vi "Command Voltages Check.vi"() -> ()   [LabVIEW 2009]
uses:
  lib/Apps/On Off Button.ctl
  lib/Calibration/Command Voltage Check Ramp States.ctl
  Test Utilities/DAQ Read Actions.ctl
  <vilib>/DAQmx/write.llb/DAQmx Write (Analog 1D DBL NChan 1Samp).vi
  Program Files (x86)/National Instruments/LabVIEW 2009/resource/objmgr/daqmx.rc
panel:
  in  "error out":errorcluster
  out "Cmd Volt Chk Ramp States":T1
  in  "Ramping":T2
  in  "Number of\nIntervals":i32
  in  "Half Period (msec)":i32
  in  "Peak Value":dbl
  in  "Offset":dbl
  out "Diffs":dbl[](array[numeric])=[-7.680882880270997, -8.566659800159199, -9.658116593296763, -9.594949810916727, -8.940447035067507, -8.192445315897492] format="%^#_10g"
  out "Write error out":errorcluster
  out "Monitor":dbl[](array[numeric])=[-7.680882880270997, -8.566659800159199, -9.658116593296763, -9.594949810916727, -8.940447035067507, -8.192445315897492] format="%^#_10g"
  out "Command \nVoltage":dbl[](array[numeric])=[-0.0, -0.0, -0.0, -0.0, -0.0, -0.0] format="%^#_10g"
  out "Control Voltage":dbl[](array[numeric])=[-0.0, -0.0, -0.0, -0.0, -0.0, -0.0]
  in  "Quit":bool
  in  "rate":dbl=100.0
  in  "samples per \nchannel":i32=30 caption="samples per channel"
  in  "Command Voltage Task":refnum<k21>="Command Voltage"
  in  "Monitor Task":refnum<k21>="All Readings"
  in  "Actuator":i32(listbox)
  out "Command \nVoltages":T3(graph)={"Average[0]"=-7.17251209904047, "Average[1]"=-8.19396103384171, "Average[2]"=-9.68369051887908, "Average[3]"=-9.45574535938537, "Average[4]"=-9.241187346298316, "Average[5]"=-8.612741694704903, "Average[6]"=0.0, "Average[7]"=0.0, "Average[8]"=0.0}
  out "Monitor":T3(graph)={"Average[0]"=-7.17251209904047, "Average[1]"=-8.19396103384171, "Average[2]"=-9.68369051887908, "Average[3]"=-9.45574535938537, "Average[4]"=-9.241187346298316, "Average[5]"=-8.612741694704903, "Average[6]"=0.0, "Average[7]"=0.0, "Average[8]"=0.0}
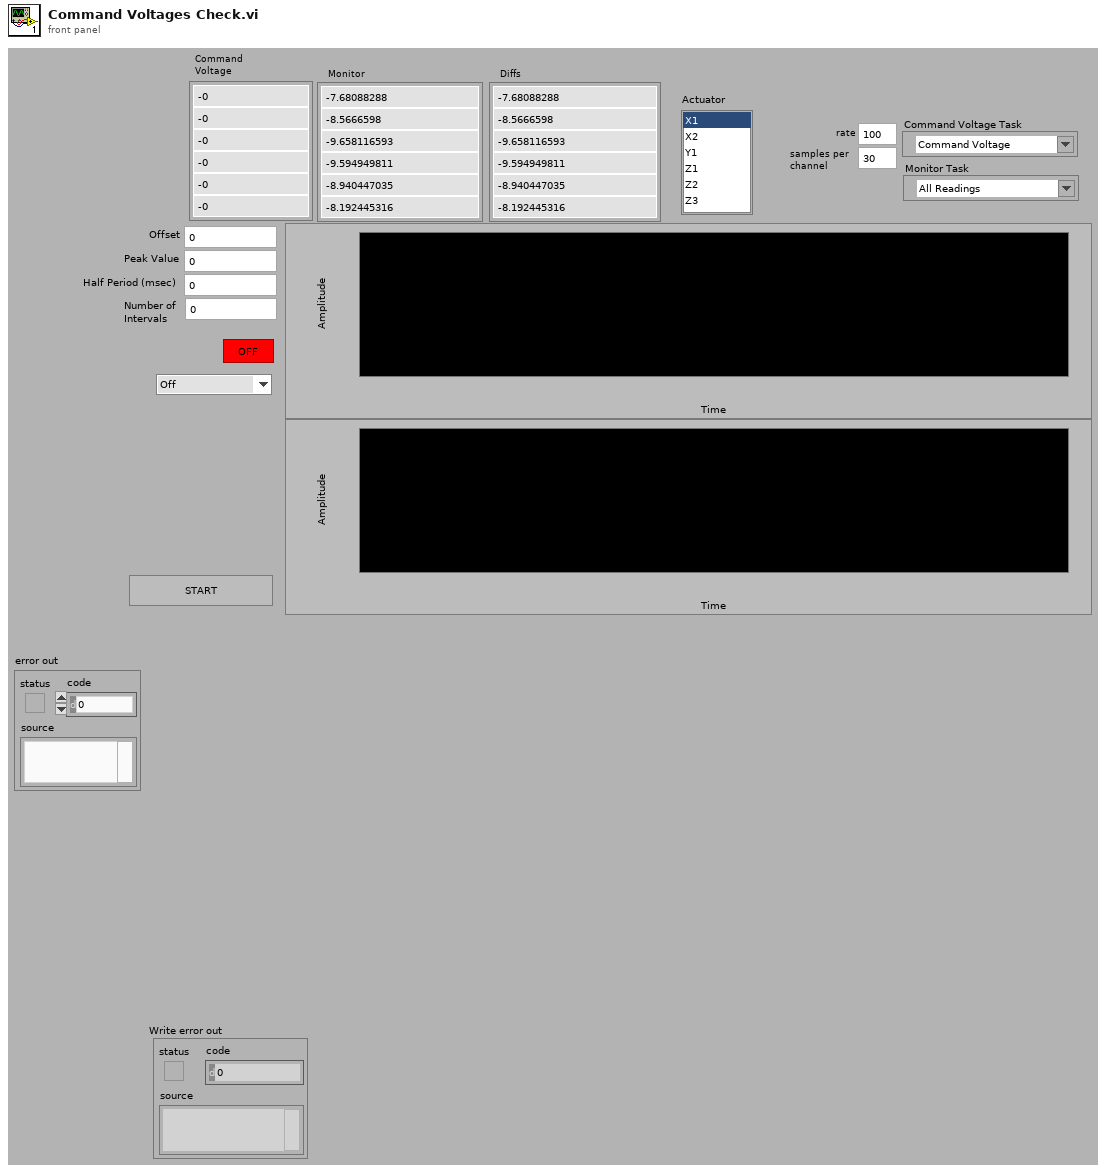
[diagram p1: front panel]
types:
  T1 = typedef "Command Voltage Check Ramp States.ctl" = enum16{"Off", "Start", "Ramp Up", "Ramp Down", "Stop"}
  T2 = typedef "On Off Button.ctl" = bool
  T3 = cluster{"Average[0]":dbl, "Average[1]":dbl, "Average[2]":dbl, "Average[3]":dbl, "Average[4]":dbl, "Average[5]":dbl, "Average[6]":dbl, "Average[7]":dbl, "Average[8]":dbl}
  T4 = typedef "DAQ Read Actions.ctl" = enum16{"Start", "Read", "Stop"}
  T5 = cluster{"Control Voltage[0]":dbl, "Control Voltage[1]":dbl, "Control Voltage[2]":dbl, "Control Voltage[3]":dbl, "Control Voltage[4]":dbl, "Control Voltage[5]":dbl, "Control Voltage[6]":dbl, "Control Voltage[7]":dbl, "Control Voltage[8]":dbl}
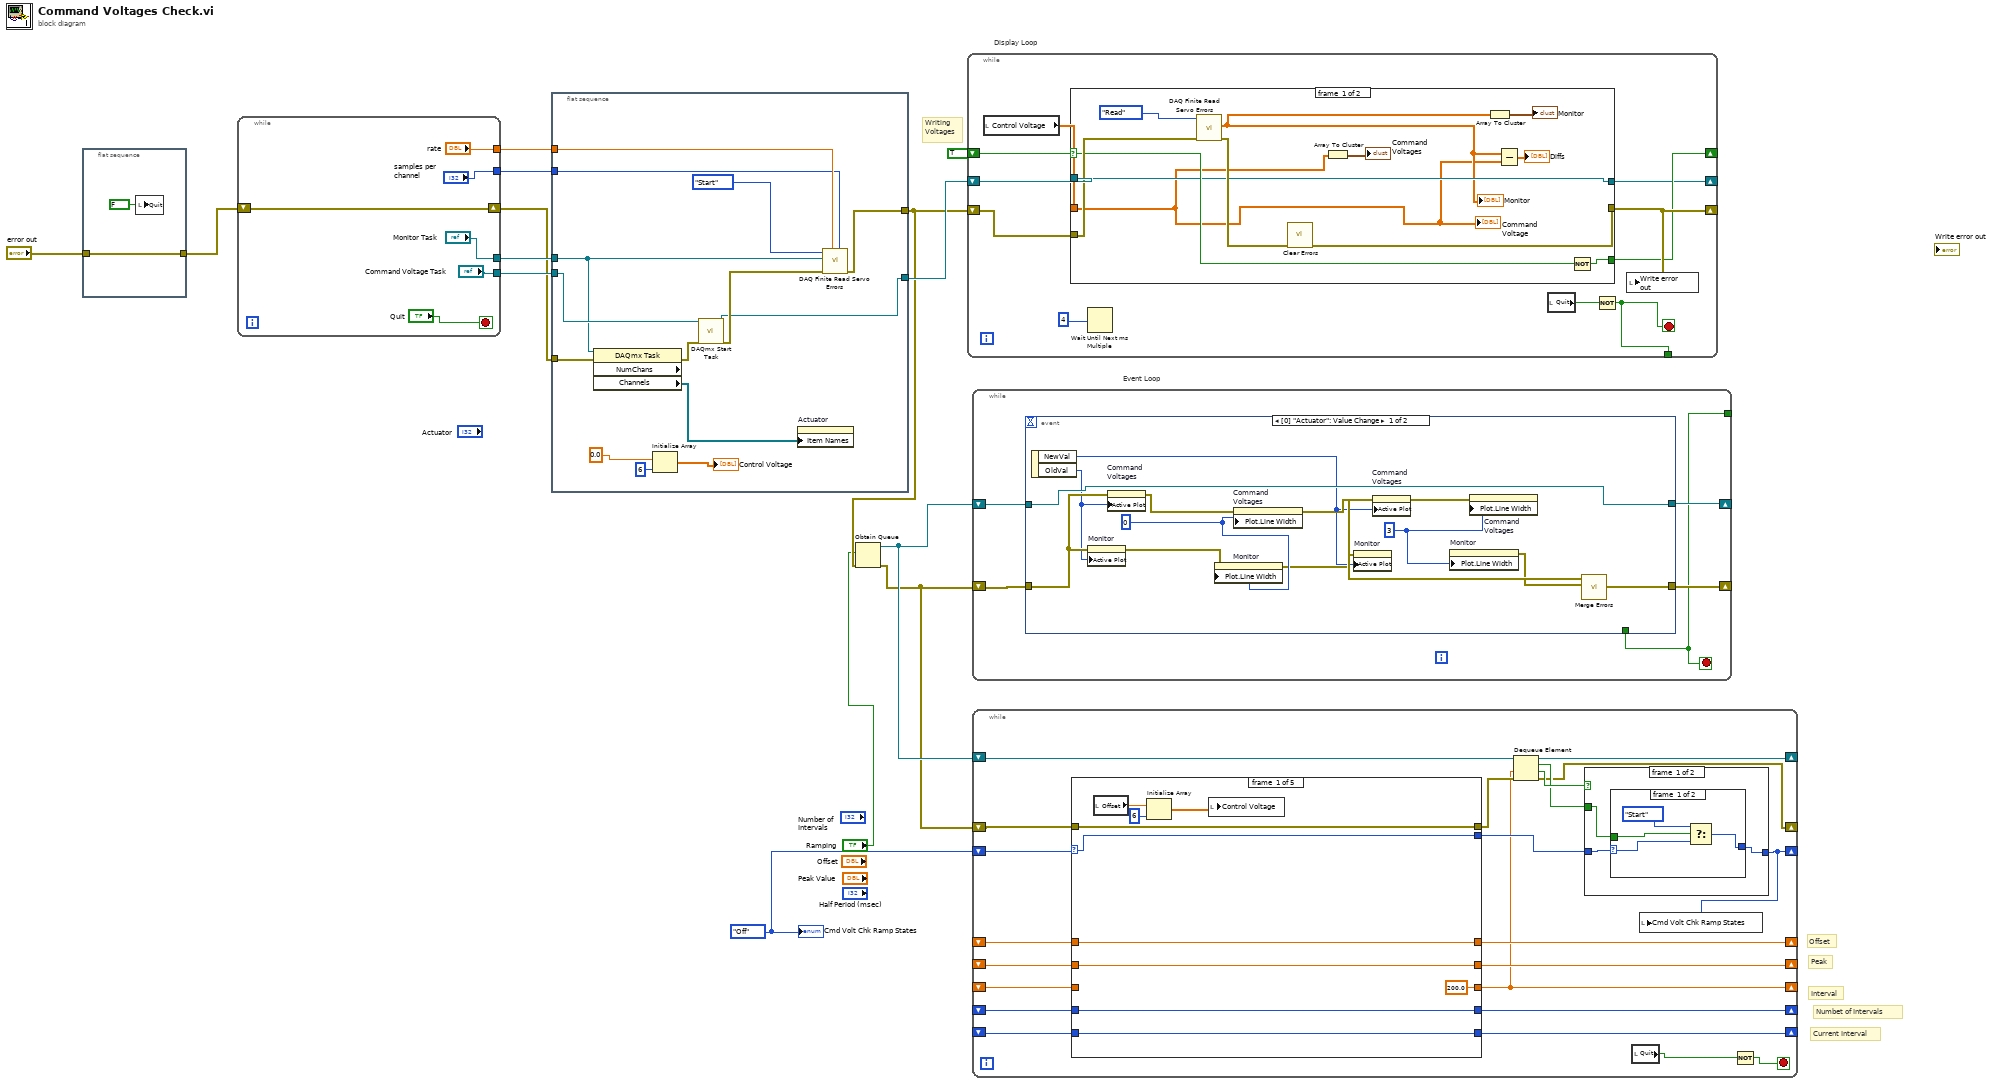
[diagram p0: block diagram]
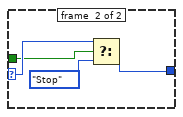
[diagram p2: hidden frame]
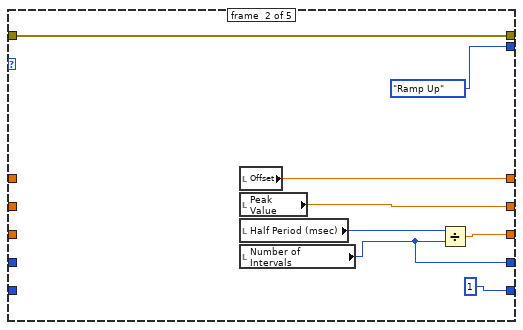
[diagram p4: hidden frame]
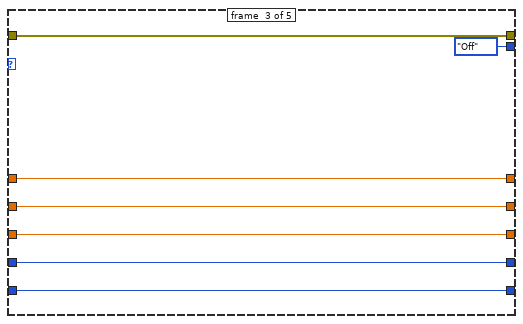
[diagram p5: hidden frame]
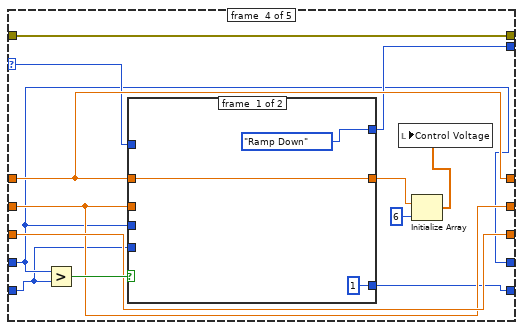
[diagram p6: hidden frame]
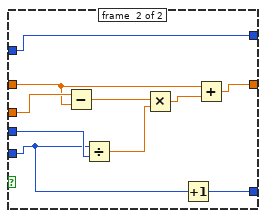
[diagram p7: hidden frame]
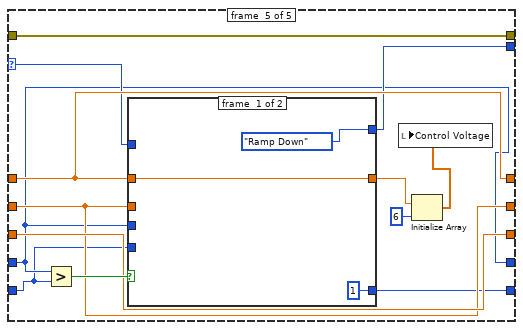
[diagram p8: hidden frame]
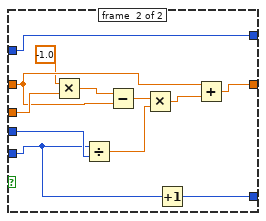
[diagram p9: hidden frame]
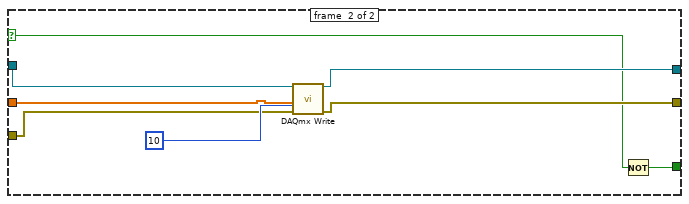
[diagram p10: hidden frame]
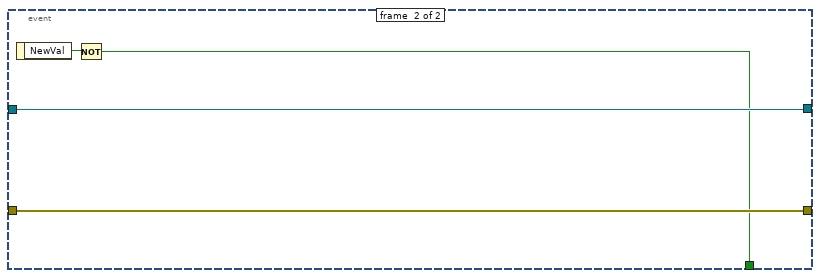
[diagram p11: hidden frame]
diagram:
  w8 = Command_Voltage_Check_Ramp_States."Off" ("Cmd Volt Chk Ramp States")
  # "Current Interval"
  # "Numbet of Intervals"
  # "Interval"
  # "Peak"
  # "Offset"
  # "Writing\nVoltages"
  n1 = flat-sequence {
    tunnel: "error out" -> [w16]
    tunnel: [w16] -> w1
    frame #0 {
      n2 = local write "Quit"(FALSE ("Quit")) -> ()
    }
  }
  n3 = while {
    tunnel: ["Command Voltage Task"] -> w14
    tunnel: ["Monitor Task"] -> w13
    tunnel: ["rate"] -> w12
    tunnel: ["samples per \nchannel"] -> w11
    shift-right: [w17] -> w3
    shift-left: w1 -> [w17]
    stop <- "Quit" stop-if-true
  }
  n4 = flat-sequence {
    tunnel: w14 -> [w35]
    tunnel: w13 -> [w26]
    tunnel: w12 -> [w34]
    tunnel: w11 -> [w33]
    tunnel: [w28] -> w7
    tunnel: [w27] -> w10
    tunnel: w3 -> [w23]
    frame #0 {
      n5 = property class="DAQmx Task" props=["NumChans", "Channels"](reference=w26, error in=w23) -> (error out=w25:errorcluster, "Channels"=w24:refnum<k21>[])  [unwired: 2 out]
      n6 = Initialize Array(0.0, 6 ("dimension size")) -> (→"Control Voltage":dbl[])
      n7 = call <vilib>:"DAQmx Start Task.vi"("task/channels in"=w35, "error in"=w25) -> ("task out"=w27:refnum<k21>, "error out"=w29:errorcluster)  [unwired: 12 out]
      n8 = property on="Actuator" class="LstBox (strict)"("Item Names"=w24) -> ()  [unwired: 2 in, 2 out]
      n9 = call "DAQ Finite Read Servo Errors.vi"("samples per channel"=w33, "rate"=w34, "error in"=w29, "task/channels in"=w26, "Action"=DAQ_Read_Actions."Start") -> ("error out"=w28:errorcluster)  [unwired: 6 out]
    }
  }
  n10 = Obtain Queue(element data type="Ramping", error in (no error)=w7) -> (queue out=w6:refnum<queue>, error out=w4:errorcluster)  [unwired: 3 in, 1 out]
  n11 = while "Display Loop" {
    shift-right: [w41] -> _
    shift-left: w7 -> [w42]
    tunnel: [w44] -> _
    shift-right: [w40] -> _
    shift-left: TRUE -> [w39]
    shift-right: [w37] -> _
    shift-left: w10 -> [w38]
    stop <- w44 stop-if-true
    n12 = local read "Control Voltage"() -> (w43:dbl[])
    n13 = case shown="True" w39 {
      selector: w39 -> [w52 w59]
      tunnel: w43 -> [w47 w62]
      tunnel: w42 -> [w55 w64]
      tunnel: [w53 w63] -> w41
      tunnel: [w51 w60] -> w40
      tunnel: w38 -> [w50 w65]
      tunnel: [w50 w61] -> w37
      frame #0 {
        n14 = call "DAQ Finite Read Servo Errors.vi"("error in"=w55, "Action"=DAQ_Read_Actions."Read") -> ("error out"=w54:errorcluster, "Average"=w48:dbl[])  [unwired: 3 in, 5 out]
        "Monitor" <- w48
        n15 = call <vilib>:"Clear Errors.vi"("error in (no error)"=w54) -> ("error out"=w53:errorcluster)  [unwired: 6 out]
        n16 = Array To Cluster(array=w47) -> (cluster=→"Command \nVoltages":T5)
        n17 = Array To Cluster(array=w48) -> (cluster=→"Monitor":T3)
        n18 = Subtract(x=w48, y=w47) -> (x-y=→"Diffs":dbl[])
        n19 = Not(x=w52) -> (.not. x?=w51:bool)
        "Command \nVoltage" <- w47
      }
      frame #1 {
        n20 = call-poly <vilib>:"DAQmx Write.vi"("task/channels in"=w65, "data"=w62, "timeout"=10, "error in"=w64) -> ("task out"=w61:refnum<k21>, "error out"=w63:errorcluster)  [unwired: 1 in, 9 out]
        n21 = Not(x=w59) -> (.not. x?=w60:bool)
      }
    }
    n22 = Wait Until Next ms Multiple(millisecond multiple=4) -> ()  [unwired: 1 out]
    n23 = local read "Quit"() -> (w45:bool)
    n24 = Not(x=w45) -> (.not. x?=w44:bool)
    n25 = local write "Write error out"(w41) -> ()
  }
  n26 = while "Event Loop" {
    tunnel: [w67] -> _
    shift-right: [w68] -> _
    shift-left: w4 -> [w70]
    shift-right: [w69] -> _
    shift-left: w6 -> [w71]
    stop <- w67 stop-if-true
    n27 = event shown="[0] \"Actuator\": Value Change" {
      selector: _ -> [_ _]
      dyn-events: _ -> [_ _]
      timeout: _ -> [_ _]
      tunnel: w71 -> [w81 w88]
      tunnel: w70 -> [w80 w89]
      tunnel: [w81 w88] -> w69
      tunnel: [w73 w89] -> w68
      tunnel: [_ w86] -> w67
      event #0 {
        w74 = u8 3 ("Plot.Line Width")
        w78 = u8 0 ("Plot.Line Width")
        n28 = event-data() -> ("NewVal"=w75:i32, "OldVal"=w79:i32)  [unwired: 1 out]
        n29 = property on="Monitor" class="WFChart (strict)"(error in=w80, "Active Plot"=w79) -> (error out=w77:errorcluster)  [unwired: 1 in, 1 out]
        n30 = property on="Command \nVoltages" class="WFChart (strict)"(error in=w80, "Active Plot"=w79) -> (error out=w85:errorcluster)  [unwired: 1 in, 1 out]
        n31 = property on="Monitor" class="WFChart (strict)"(error in=w77, "Plot.Line Width"=w78) -> (error out=w76:errorcluster)  [unwired: 1 in, 1 out]
        n32 = property on="Command \nVoltages" class="WFChart (strict)"(error in=w85, "Plot.Line Width"=w78) -> (error out=w84:errorcluster)  [unwired: 1 in, 1 out]
        n33 = property on="Monitor" class="WFChart (strict)"(error in=w76, "Active Plot"=w75) -> ()  [unwired: 1 in, 2 out]
        n34 = property on="Command \nVoltages" class="WFChart (strict)"(error in=w84, "Active Plot"=w75) -> (error out=w83:errorcluster)  [unwired: 1 in, 1 out]
        n35 = property on="Monitor" class="WFChart (strict)"("Plot.Line Width"=w74) -> (error out=w72:errorcluster)  [unwired: 2 in, 1 out]
        n36 = property on="Command \nVoltages" class="WFChart (strict)"(error in=w83, "Plot.Line Width"=w74) -> (error out=w82:errorcluster)  [unwired: 1 in, 1 out]
        n37 = call <vilib>:"Merge Errors.vi"("error in 2 (no error)"=w72, "error in 1 (no error)"=w82) -> ("error out"=w73:errorcluster)  [unwired: 5 in]
      }
      event #1 {
        n38 = event-data() -> ("NewVal"=w87:bool)  [unwired: 1 out]
        n39 = Not(x=w87) -> (.not. x?=w86:bool)
      }
    }
  }
  n40 = while {
    shift-right: [w93] -> _
    shift-left: w8 -> [w111]
    shift-right: [w104] -> _
    shift-left: w4 -> [w110]
    shift-right: [w103] -> _
    shift-left: w6 -> [w109]
    shift-right: [w92] -> _
    shift-left: _ -> [w96]
    shift-right: [w101] -> _
    shift-left: _ -> [w97]
    shift-right: [w102] -> _
    shift-left: _ -> [w98]
    shift-right: [w100] -> _
    shift-left: _ -> [w95]
    shift-right: [w99] -> _
    shift-left: _ -> [w94]
    stop <- w91 stop-if-true
    n41 = case shown="\"Off\"" w111 {
      selector: w111 -> [w129 _ _ w153 w179]
      tunnel: w110 -> [w130 w134 w143 w161 w187]
      tunnel: [w130 w134 w143 w161 w187] -> w108
      tunnel: [w129 Command_Voltage_Check_Ramp_States."Ramp Up" ("Cmd Volt Chk Ramp States") Command_Voltage_Check_Ramp_States."Off" ("Cmd Volt Chk Ramp States") w152 w178] -> w105
      tunnel: [w128 w141 w148 w155 w181] -> w102
      tunnel: [w127 w140 w147 w154 w180] -> w101
      tunnel: [200.0 w138 w144 w159 w185] -> w92
      tunnel: [w125 w137 w146 w151 w177] -> w100
      tunnel: [w124 1 w145 w149 w175] -> w99
      tunnel: w98 -> [w128 _ w148 w155 w181]
      tunnel: w97 -> [w127 _ w147 w154 w180]
      tunnel: w96 -> [_ _ w144 w159 w185]
      tunnel: w95 -> [w125 _ w146 w151 w177]
      tunnel: w94 -> [w124 _ w145 w150 w176]
      frame #0 {
        n42 = local read "Offset"() -> (w133:dbl)
        n43 = Initialize Array(w133, 6 ("dimension size")) -> (w131:dbl[])
        n44 = local write "Control Voltage"(w131) -> ()
      }
      frame #1 {
        n45 = local read "Offset"() -> (w141:dbl)
        n46 = local read "Peak Value"() -> (w140:dbl)
        n47 = local read "Half Period (msec)"() -> (w139:i32)
        n48 = local read "Number of\nIntervals"() -> (w137:i32)
        n49 = Divide(x=w139, y=w137) -> (x/y=w138:dbl)
      }
      frame #2 {
      }
      frame #3 {
        n50 = Greater?(x=w151, y=w150) -> (0:w160:bool)
        n51 = case shown="False" w160 {
          tunnel: w154 -> [_ w170]
          tunnel: w155 -> [w164 w169]
          tunnel: [w164 w167] -> w157
          tunnel: w153 -> [_ w174]
          tunnel: [Command_Voltage_Check_Ramp_States."Ramp Down" ("Cmd Volt Chk Ramp States") w174] -> w152
          tunnel: w151 -> [_ w173]
          tunnel: w150 -> [_ w166]
          tunnel: [1 w165] -> w149
          frame #0 {
          }
          frame #1 {
            n52 = Subtract(x=w170, y=w169) -> (x-y=w172:dbl)
            n53 = Divide(x=w166, y=w173) -> (x/y=w171:dbl)
            n54 = Multiply(x=w172, y=w171) -> (x*y=w168:dbl)
            n55 = Increment(x=w166) -> (x+1=w165:i32)
            n56 = Add(x=w169, y=w168) -> (x+y=w167:dbl)
          }
        }
        n57 = Initialize Array(w157, 6 ("dimension size")) -> (w156:dbl[])
        n58 = local write "Control Voltage"(w156) -> ()
      }
      frame #4 {
        n59 = Greater?(x=w177, y=w176) -> (0:w186:bool)
        n60 = case shown="False" w186 {
          tunnel: w180 -> [_ w198]
          tunnel: w181 -> [w190 w197]
          tunnel: [w190 w195] -> w183
          tunnel: w179 -> [_ w202]
          tunnel: [Command_Voltage_Check_Ramp_States."Ramp Down" ("Cmd Volt Chk Ramp States") w202] -> w178
          tunnel: w177 -> [_ w201]
          tunnel: w176 -> [_ w192]
          tunnel: [1 w191] -> w175
          frame #0 {
          }
          frame #1 {
            n61 = Multiply(x=-1.0, y=w198) -> (x*y=w194:dbl)
            n62 = Divide(x=w192, y=w201) -> (x/y=w199:dbl)
            n63 = Subtract(x=w194, y=w197) -> (x-y=w200:dbl)
            n64 = Multiply(x=w200, y=w199) -> (x*y=w196:dbl)
            n65 = Increment(x=w192) -> (x+1=w191:i32)
            n66 = Add(x=w197, y=w196) -> (x+y=w195:dbl)
          }
        }
        n67 = Initialize Array(w183, 6 ("dimension size")) -> (w182:dbl[])
        n68 = local write "Control Voltage"(w182) -> ()
      }
    }
    n69 = Dequeue Element(queue=w109, timeout in ms (-1)=w92, error in (no error)=w108) -> (queue out=w103:refnum<queue>, element=w106:T2, timed out?=w107:bool, error out=w104:errorcluster)
    n70 = case shown="False" w107 {
      tunnel: w106 -> [w113 _]
      tunnel: w105 -> [w114 w123]
      tunnel: [w112 w123] -> w93
      frame #0 {
        n71 = case shown="\"Start\", Default" w114 {
          selector: w114 -> [w117 w122]
          tunnel: w113 -> [w118 w121]
          tunnel: [w116 w119] -> w112
          frame #0 {
            n72 = Select(t=Command_Voltage_Check_Ramp_States."Start", s=w118, f=w117) -> (s? t:f=w116:T1)
          }
          frame #1 {
            n73 = Select(t=w122, s=w121, f=Command_Voltage_Check_Ramp_States."Stop") -> (s? t:f=w119:T1)
          }
        }
      }
      frame #1 {
      }
    }
    n74 = local read "Quit"() -> (w90:bool)
    n75 = local write "Cmd Volt Chk Ramp States"(w93) -> ()
    n76 = Not(x=w90) -> (.not. x?=w91:bool)
  }
  "Cmd Volt Chk Ramp States" <- w8
